vi "pattern.vi"() -> ()   [LabVIEW 2019]
panel:
  out "Pattern":string[](array[string])
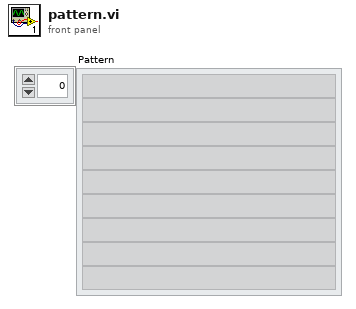
[diagram p1: front panel]
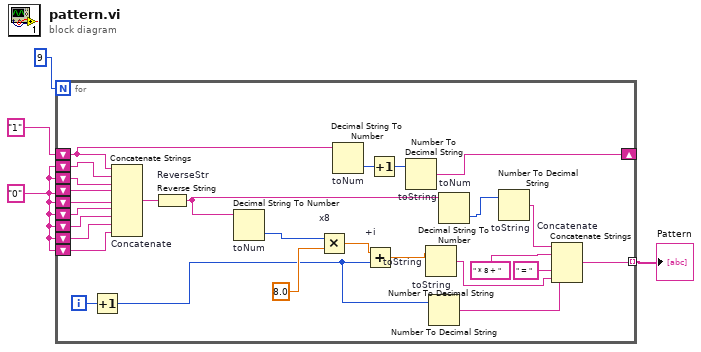
[diagram p0: block diagram]
diagram:
  w2 = "0"
  n1 = for {
    N: 9 -> [_]
    shift-right: [w16] -> _
    shift-left: "1" -> [w27]
    shift-left: w2 -> [w26]
    shift-left: w2 -> [w25]
    shift-left: w2 -> [w24]
    shift-left: w2 -> [w23]
    shift-left: w2 -> [w22]
    shift-left: w2 -> [w21]
    shift-left: w2 -> [w20]
    shift-left: w2 -> [w19]
    tunnel: [w13] -> w1 mode=indexing
    i -> [w30]
    # "Pattern"
    n2 = Increment(x=w30) -> (x+1=w11:i32)
    n3 = Concatenate Strings "Concatenate"(w27, w26, w25, w24, w23, w22, w21, w20, w19) -> (w15:string)
    n4 = Reverse String "ReverseStr"(1:w15) -> (0:w5:string)
    n5 = Decimal String To Number "toNum"(string=w5) -> (number=w17:i32)  [unwired: 2 in, 1 out]
    n6 = Multiply "x8"(x=w17, y=8.0) -> (x*y=w18:dbl)
    n7 = Decimal String To Number "toNum"(string=w27) -> (number=w29:i32)  [unwired: 2 in, 1 out]
    n8 = Add "+i"(x=w18, y=w11) -> (x+y=w14:dbl)
    n9 = Increment(x=w29) -> (x+1=w28:i32)
    n10 = Number To Decimal String "toString"(number=w28) -> (decimal integer string=w16:string)  [unwired: 1 in]
    n11 = Number To Decimal String "toString"(number=w14) -> (decimal integer string=w8:string)  [unwired: 1 in]
    n12 = Number To Decimal String "toString"(number=w11) -> (decimal integer string=w10:string)  [unwired: 1 in]
    n13 = Decimal String To Number "toNum"(string=w5) -> (number=w6:i32)  [unwired: 2 in, 1 out]
    n14 = Number To Decimal String "toString"(number=w6) -> (decimal integer string=w7:string)  [unwired: 1 in]
    n15 = Concatenate Strings "Concatenate"(w7, " * 8 + " ("string"), w10, " = " ("string"), w8) -> (w13:string)
  }
  "Pattern" <- w1
